vi "Swift.destructor.vi"(0 "i ref in":refnum<vi>, 5 "error in(no error)":errorcluster) -> (19 "error out":errorcluster)   [LabVIEW 2014, in "Swift.lvlib"]
doc: "This is the destructor of a class.\n\nLicense Agreement for this software:\n\nCopyright (C)\nGesellschaft für Schwerionenforschung, GSI\nPlanckstr. 1\n64291 Darmstadt\nGermany\n\nContact: D.Beck@gsi.de \n\nThis program is free software; you can redistribute it and/or modify it under the terms of the \nGNU General Public License as published by the Free Software Foundation; either version 2 of \nthe license, or (at your option) any later version.\n\nThis program is distributed in the hope that it will be useful, but WITHOUT ANY WARRANTY; \nwithout even the implied warranty of MERCHANTABILITY or FITNESS FOR A PARTICULAR PURPOSE. See the GNU General License for more details (http://www.gnu.org).\n\nGesellschaft für Schwerionenforschung, GSI\nPlanckstr. 1, 64291 Darmstadt, Germany\nFor all questions and ideas contact: M.Richter@gsi.de, H.Brand@gsi.de or D.Beck@gsi.de.\nLast update: 16-JUN-2004"
uses:
  Swift.lvlib
  CS_Core/CSSystem/CoreLib/CoreLib.string 2 byte array.vi
  CS_Core/BaseProcess/BaseProcess.lvlib
  CS_Core/CSSystem/CSSystemLib/CSSystemLib.lvlib
  CS_Core/CSSystem/CoreLib/CoreLib.lvlib
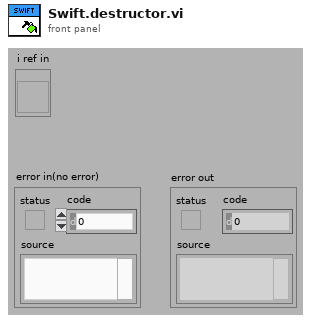
[diagram p1: front panel]
types:
  T1 = enum16{"SetAttribute", "GetAttribute", "CreateAttribute", "DestroyAttribute", "DestroyAllAtributes"}
  T2 = typedef "Swift.lvlib/Swift.i attribute.ctl" = cluster{"SWIFT Frequency Generator":string}
  T3 = typedef "CoreDefs.rawDataType.ctl" = i8[]
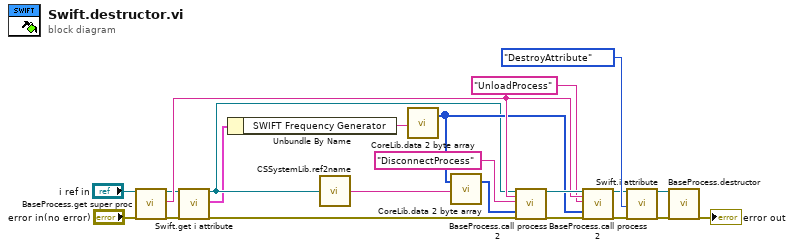
[diagram p0: block diagram]
diagram:
  n1 = call "BaseProcess.get super proc.vi"("i ref in"="i ref in", "error in (no error)"="error in(no error)") -> ("i ref out"=w11:refnum<vi>, "SuperProc"=w14:string, "error out"=w4:errorcluster)  [unwired: 15 in]
  n2 = call "Swift.get i attribute.vi"("i ref in"=w11, "error in (no error)"=w4) -> ("i ref out"=w10:refnum<vi>, "CLASS.i attribute out"=w9:T2, "error out"=w3:errorcluster)  [unwired: 15 in]
  n3 = Unbundle By Name(w9) -> ("SWIFT Frequency Generator"=w8:string)
  n4 = call "CSSystemLib.ref2name.vi"("obj refnum"=w10) -> ("name"=w17:string)
  n5 = call-poly "CoreLib.data 2 byte array.vi"("string"=w8) -> ("byteArray out"=w12:T3)  [unwired: 18 in]
  n6 = call-poly "CoreLib.data 2 byte array.vi"("byteArray"=w12, "string"=w17) -> ("byteArray out"=w16:T3)  [unwired: 17 in]
  n7 = call "BaseProcess.call process 2.vi"("i ref in"=w10, "Object"=w14, "Selector"="DisconnectProcess", "Data"=w16, "error in (no error)"=w3) -> ("i ref out"=w15:refnum<vi>, "error out"=w2:errorcluster)  [unwired: 13 in]
  n8 = call "BaseProcess.call process 2.vi"("i ref in"=w15, "Object"=w14, "Selector"="UnloadProcess", "Data"=w12, "error in (no error)"=w2) -> ("i ref out"=w6:refnum<vi>, "error out"=w1:errorcluster)  [unwired: 13 in]
  n9 = call "Swift.i attribute.vi"("VI Refnum"=w6, "Action"=T1."DestroyAttribute", "error in (no error)"=w1) -> ("VI Refnum out"=w21:refnum<vi>, "error out"=w20:errorcluster)  [unwired: 14 in, 1 out]
  n10 = call "BaseProcess.destructor.vi"("i ref in"=w21, "error in (no error)"=w20) -> ("error out"=→"error out":errorcluster)  [unwired: 17 in]
